vi "Main.vi"   [LabVIEW 2014]
uses:
  Class/RealSubject1/RealSubject1.lvclass
  Class/Subject/Subject.lvclass
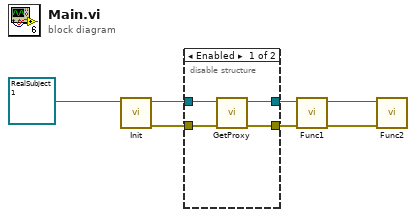
[diagram p0: block diagram]
diagram:
  n1 = call-dynamic "Init.vi"("RealSubject1 in"=refnum<class "RealSubject1.lvclass"> refnum ("forcible Proxy.lvlib:RealSubject1")) -> ("error out"=w3:errorcluster, "RealSubject1 out"=w4:refnum<class "RealSubject1.lvclass">)  [unwired: 9 in]
  n2 = disable-structure shown="Enabled" {
    disable-tunnel: w4 -> [w11 w13]
    disable-tunnel: w3 -> [w10 w12]
    disable-tunnel: [w9 w12] -> w2
    disable-tunnel: [w8 w13] -> w1
    frame Enabled {
      n3 = call "GetProxy.vi"("error in (no error)"=w10, "Subject in"=w11) -> ("error out"=w9:errorcluster, "Proxy"=w8:refnum<class "Subject.lvclass">)  [unwired: 8 in]
    }
    frame Disabled {
    }
  }
  n4 = call-dynamic "Func1.vi"("error in (no error)"=w2, "Subject in"=w1) -> ("error out"=w5:errorcluster, "Subject out"=w6:refnum<class "Subject.lvclass">)  [unwired: 8 in]
  n5 = call-dynamic "Func2.vi"("error in (no error)"=w5, "Subject in"=w6) -> ()  [unwired: 8 in, 2 out]
